vi "temperature_decluster_by_time.vi"(9 "t_final":dbl format="%_19f", 10 "t_init":dbl format="%_19f", 11 "temperature array cluster":T1) -> (2 "Dados":dbl[][](array[numeric]), 3 "Tempo":dbl[](array[numeric]))   [LabVIEW 2019]
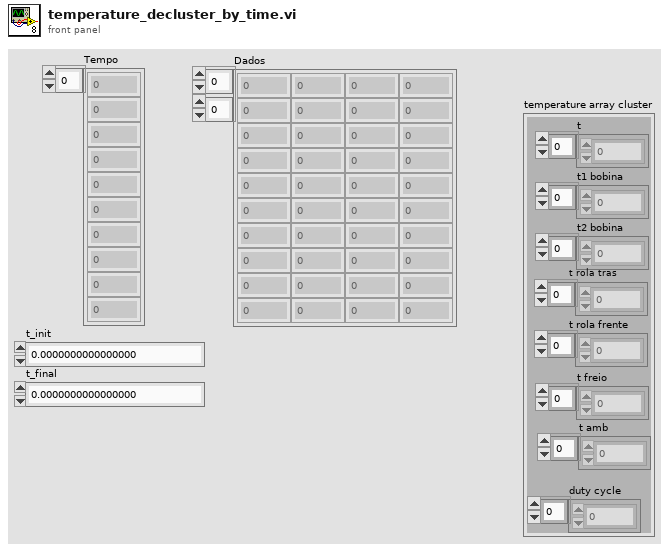
[diagram p1: front panel]
types:
  T1 = cluster{"t":dbl[], "t1 bobina":dbl[], "t2 bobina":dbl[], "t freio":dbl[], "t rola frente":dbl[], "t rola tras":dbl[], "t amb":dbl[], "duty cycle":dbl[]}
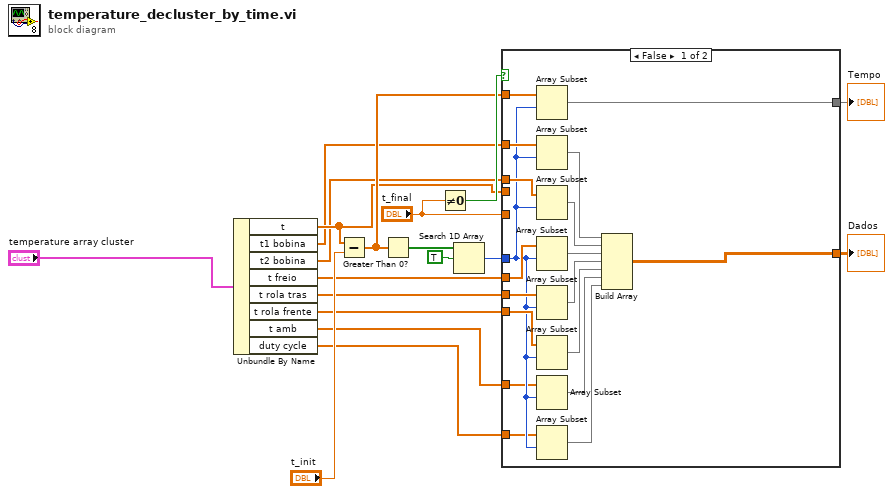
[diagram p0: block diagram]
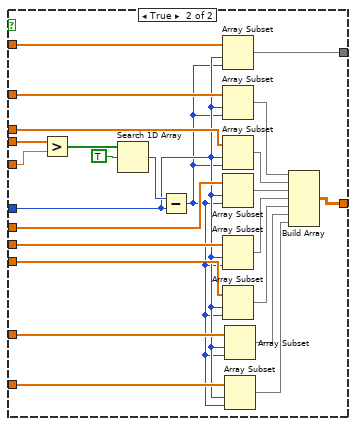
[diagram p2: hidden frame]
diagram:
  n1 = Unbundle By Name("temperature array cluster") -> ("t"=w13:dbl[], "t1 bobina"=w8:dbl[], "t2 bobina"=w9:dbl[], "t freio"=w10:dbl[], "t rola tras"=w5:dbl[], "t rola frente"=w4:dbl[], "t amb"=w2:dbl[], "duty cycle"=w1:dbl[])
  n2 = Subtract(x=w13, y="t_init") -> (x-y=w15:dbl[])
  n3 = Greater Than 0?(x=w15) -> (x > 0?=w17:bool[])
  n4 = Not Equal To 0?(x="t_final") -> (x != 0?=w16:bool)
  n5 = Search 1D Array(1D array=w17, element=TRUE) -> (index of element=w14:i32)  [unwired: 1 in]
  n6 = case shown="False" w16 {
    tunnel: w15 -> [w36 w60]
    tunnel: w14 -> [w23 w38]
    tunnel: [w35 w59] -> w7
    tunnel: "t_final" -> [_ w55]
    tunnel: w13 -> [_ w54]
    tunnel: w10 -> [w31 w49]
    tunnel: w9 -> [w30 w50]
    tunnel: w8 -> [w29 w51]
    tunnel: [w28 w48] -> w6
    tunnel: w5 -> [w25 w46]
    tunnel: w4 -> [w24 w45]
    tunnel: w2 -> [w22 w41]
    tunnel: w1 -> [w21 w39]
    frame False {
      n7 = Array Subset(array=w36, index=w23) -> (w35:dbl[])  [unwired: 1 in]
      n8 = Array Subset(array=w29, index=w23) -> (w32:dbl[])  [unwired: 1 in]
      n9 = Array Subset(array=w30, index=w23) -> (w33:dbl[])  [unwired: 1 in]
      n10 = Array Subset(array=w31, index=w23) -> (w34:dbl[])  [unwired: 1 in]
      n11 = Array Subset(array=w25, index=w23) -> (w27:dbl[])  [unwired: 1 in]
      n12 = Array Subset(array=w24, index=w23) -> (w26:dbl[])  [unwired: 1 in]
      n13 = Array Subset(array=w22, index=w23) -> (w20:dbl[])  [unwired: 1 in]
      n14 = Array Subset(array=w21, index=w23) -> (w19:dbl[])  [unwired: 1 in]
      n15 = Build Array(w32, w33, w34, w27, w26, w20, w19) -> (w28:dbl[][])
    }
    frame True {
      n16 = Greater?(x=w54, y=w55) -> (0:w57:bool[])
      n17 = Search 1D Array(1D array=w57, element=TRUE) -> (index of element=w58:i32)  [unwired: 1 in]
      n18 = Subtract(x=w58, y=w38) -> (x-y=w37:i32)
      n19 = Array Subset(array=w60, index=w38, length=w37) -> (w59:dbl[])
      n20 = Array Subset(array=w51, index=w38, length=w37) -> (w52:dbl[])
      n21 = Array Subset(array=w50, index=w38, length=w37) -> (w53:dbl[])
      n22 = Array Subset(array=w49, index=w38, length=w37) -> (w47:dbl[])
      n23 = Array Subset(array=w46, index=w38, length=w37) -> (w44:dbl[])
      n24 = Array Subset(array=w45, index=w38, length=w37) -> (w43:dbl[])
      n25 = Array Subset(array=w41, index=w38, length=w37) -> (w42:dbl[])
      n26 = Array Subset(array=w39, index=w38, length=w37) -> (w40:dbl[])
      n27 = Build Array(w52, w53, w47, w44, w43, w42, w40) -> (w48:dbl[][])
    }
  }
  "Tempo" <- w7
  "Dados" <- w6
